vi "Temp meas sim.vi"(11 "error in":errorcluster) -> (8 "Temp (deg C)":dbl=25.498185640690767 format="%.2f", 15 "error out":errorcluster)   [LabVIEW 2016]
doc: "This VI manages the temp meas via the thermal simulator\n\nPaul K Dixon\nPhysics 350\nCSUSB Physics"
uses:
  therm sim/therm sim kernel/globals/therm sim globals.vi
panel:
  # "Thermistor Temp Meas"
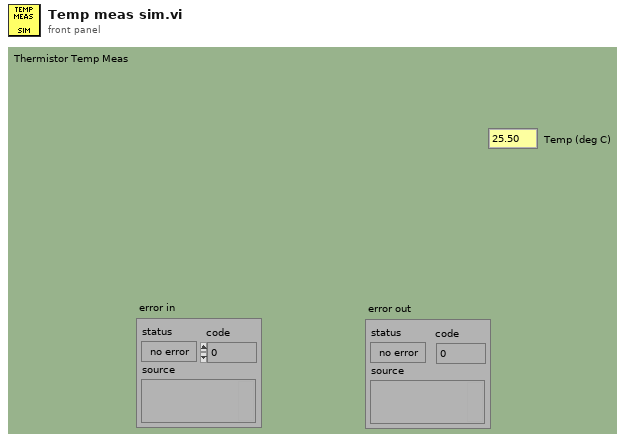
[diagram p1: front panel]
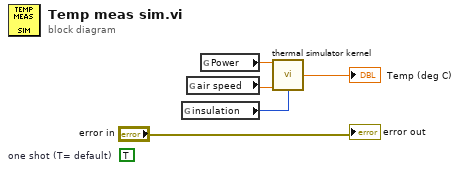
[diagram p0: block diagram]
diagram:
  (unwired) TRUE  # one shot (T= default)
  n1 = global read "therm sim globals.vi" "insulation"() -> (w1:enum16{"uncovered", "covered"})
  n2 = global read "therm sim globals.vi" "air speed"() -> (w2:dbl)
  n3 = global read "therm sim globals.vi" "Power"() -> (w3:dbl)
  n4 = call "thermal simulator kernel.vi"("Power"=w3, "air speed"=w2, "insulation"=w1) -> ("Temp"=→"Temp (deg C)":dbl)  [unwired: 11 in, 1 out]
  "error out" <- "error in"
